vi "数据上传C002.vi"(1 "数据数组":string[](array[string]), 2 "合格C002":bool) -> ()   [LabVIEW 2013]
panel:
  out "error out 2":errorcluster
  out "Result":string
  in  "error in (no error)":errorcluster
  out "error out":errorcluster
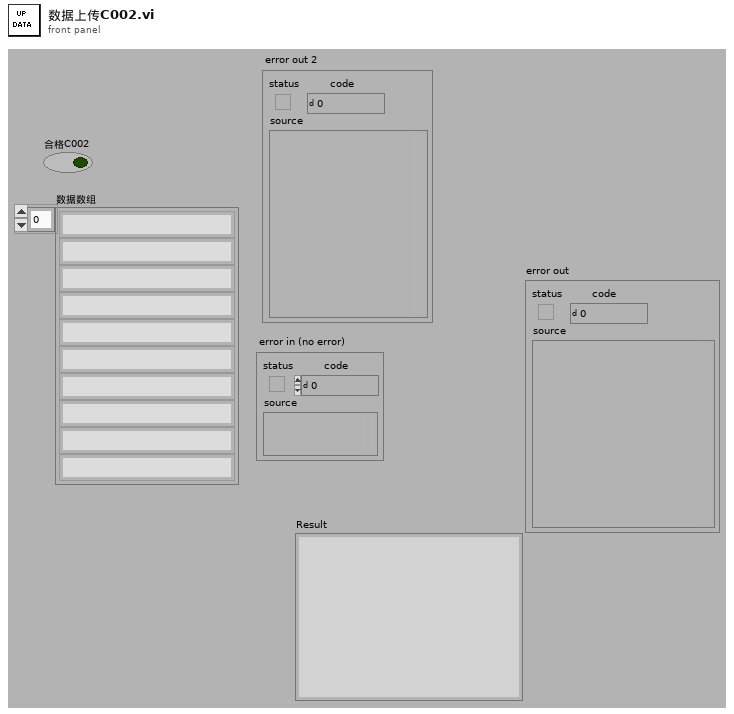
[diagram p1: front panel]
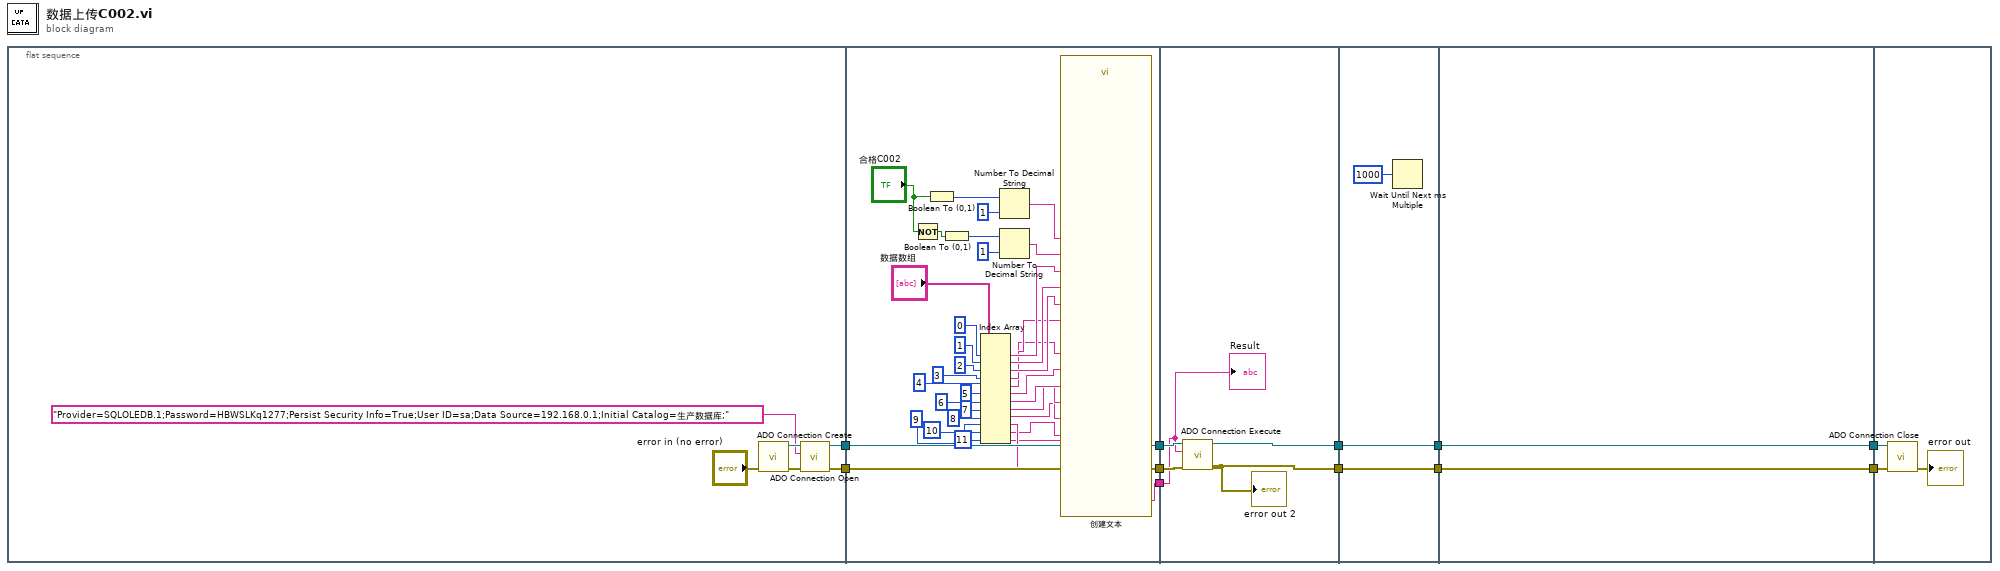
[diagram p0: block diagram]
diagram:
  n1 = flat-sequence {
    tunnel: [w13] -> w11
    tunnel: [w14] -> w10
    tunnel: w11 -> [w47]
    tunnel: w10 -> [w48]
    tunnel: [w48] -> w5
    tunnel: [w47] -> w3
    tunnel: [w39] -> w1
    tunnel: w5 -> [w58]
    tunnel: [w55] -> w4
    tunnel: w3 -> [w57]
    tunnel: [w56] -> w2
    tunnel: w1 -> [w54]
    tunnel: w4 -> [w61]
    tunnel: [w61] -> w9
    tunnel: w2 -> [w60]
    tunnel: [w60] -> w8
    tunnel: w9 -> [w62]
    tunnel: w8 -> [w63]
    tunnel: [w62] -> w7
    tunnel: [w63] -> w6
    tunnel: w7 -> [w65]
    tunnel: w6 -> [w64]
    frame #0 {
      n2 = call "ADO Connection Create.vi"("error in (no error)"="error in (no error)") -> ("error out"=w16:errorcluster, "ADODB._Connection Out"=w15:refnum<k7>)  [unwired: 9 out]
      n3 = call "ADO Connection Open.vi"("error in (no error)"=w16, "ConnectionString"="Provider=SQLOLEDB.1;Password=HBWSLKq1277;Persist Security Info=True;User ID=sa;Data Source=192.168.0.1;Initial Catalog=生产数据库;" ("字符串 2"), "ADODB._Connection In"=w15) -> ("error out"=w13:errorcluster, "ADODB._Connection Out"=w14:refnum<k7>)  [unwired: 7 out]
    }
    frame #1 {
      n4 = Not(x="合格C002") -> (.not. x?=w41:bool)
      n5 = Boolean To (0,1)(Boolean="合格C002") -> (0, 1=w53:i16)
      n6 = Boolean To (0,1)(Boolean=w41) -> (0, 1=w40:i16)
      n7 = Index Array(array="数据数组", index #1=0 ("索引"), index #2=1 ("索引"), index #3=2 ("索引"), index #4=3 ("索引"), index #5=4 ("索引"), index #6=5 ("索引"), index #7=6 ("索引"), index #8=7 ("索引"), index #9=8 ("索引"), index #10=9 ("索引"), index #11=10 ("索引"), index #12=11 ("索引")) -> (element #1=w36:string, element #2=w35:string, element #3=w34:string, element #4=w33:string, element #5=w32:string, element #6=w31:string, element #7=w30:string, element #8=w29:string, element #9=w28:string, element #10=w27:string, element #11=w26:string, element #12=w25:string)
      n8 = Number To Decimal String(number=w53, width (-)=i16 1 ("宽度(-)")) -> (decimal integer string=w38:string)
      n9 = Number To Decimal String(number=w40, width (-)=i16 1 ("宽度(-)")) -> (decimal integer string=w37:string)
      n10 = call "创建文本"("本序合格"=w38, "本序不合格"=w37, "拧紧扭矩"=w36, "拧紧角度"=w35, "拧紧合格"=w34, "拧紧不合格"=w33, "间隙值"=w32, "间隙合格"=w31, "间隙不合格"=w30, "压铆压力"=w29, "压铆合格"=w28, "压铆不合格"=w27, "员工ID"=w26, "结束时间"=w25) -> ("Result"=w39:string)  [unwired: 12 in, 1 out]
    }
    frame #2 {
      n11 = call "ADO Connection Execute.vi"("error in (no error)"=w57, "CommandText"=w54, "ADODB._Connection In"=w58) -> ("error out"=w56:errorcluster, "ADODB._Connection Out"=w55:refnum<k7>)  [unwired: 7 out]
      "error out 2" <- w56
      "Result" <- w54
    }
    frame #3 {
      n12 = Wait Until Next ms Multiple(millisecond multiple=u32 1000 ("毫秒倍数")) -> ()  [unwired: 1 out]
    }
    frame #4 {
    }
    frame #5 {
      n13 = call "ADO Connection Close.vi"("error in (no error)"=w64, "ADODB._Connection In"=w65) -> ("error out"=→"error out":errorcluster)  [unwired: 9 out]
    }
  }
